vi "Pre-Actor.vi"(8 "error in":errorcluster, 11 "DIG_IO in":refnum<class "DIG_IO.lvclass">) -> (0 "error out":errorcluster, 3 "DIG_IO out":refnum<class "DIG_IO.lvclass">)   [LabVIEW 2019, in "DIG_IO.lvlib" / "DIG_IO.lvclass"]
doc: "This override VI is to provide the means for children classes to perform application specific post launch initialization functions that must be performed *prior* to calling the actor."
uses:
  Library/DIG_IO.lvclass
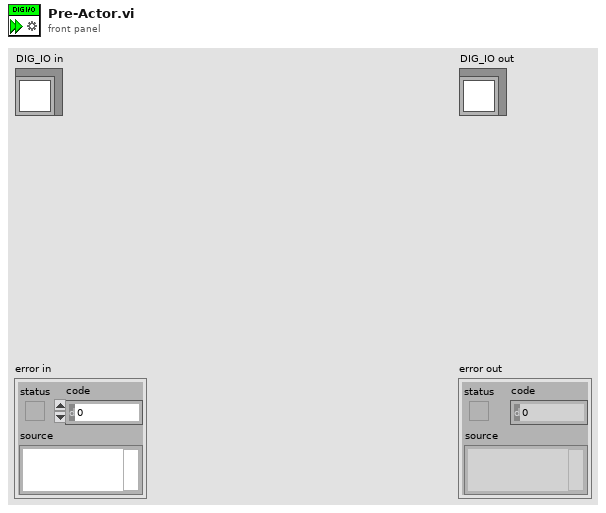
[diagram p1: front panel]
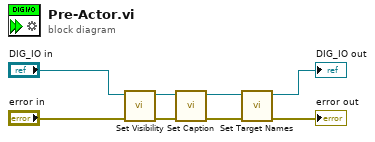
[diagram p0: block diagram]
diagram:
  n1 = call "Set Visibility.vi"("error in"="error in", "DIG_IO in"="DIG_IO in") -> ("error out"=w5:errorcluster, "DIG_IO out"=w6:refnum<class "DIG_IO.lvclass">)  [unwired: 8 in]
  n2 = call "Set Caption.vi"("error in"=w5, "DIG_IO in"=w6) -> ("error out"=w3:errorcluster, "DIG_IO out"=w4:refnum<class "DIG_IO.lvclass">)  [unwired: 8 in]
  n3 = call "Set Target Names.vi"("error in"=w3, "DIG_IO in"=w4) -> ("error out"=→"error out":errorcluster, "DIG_IO out"=→"DIG_IO out":refnum<class "DIG_IO.lvclass">)  [unwired: 8 in]
